vi "SubtractPolarVectors.vi"(10 "B":cluster{"Magnitude":dbl, "Direction":dbl}, 11 "A":cluster{"Magnitude":dbl, "Direction":dbl}) -> (3 "A-B":cluster{"Magnitude":dbl, "Direction":dbl})   [LabVIEW 2014]
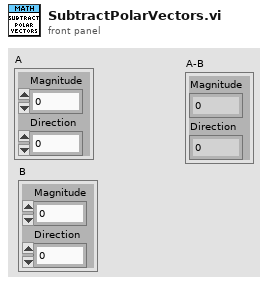
[diagram p1: front panel]
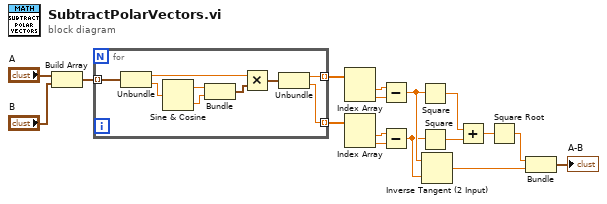
[diagram p0: block diagram]
diagram:
  n1 = Build Array("A", "B") -> (w15:cluster{"Magnitude":dbl, "Direction":dbl}[])
  n2 = for {
    tunnel: w15 -> [w26] mode=indexing
    tunnel: [w19] -> w14 mode=indexing
    tunnel: [w18] -> w13 mode=indexing
    n3 = Unbundle(w26) -> ("Magnitude"=w21:dbl, "Direction"=w25:dbl)
    n4 = Sine & Cosine(0:w25) -> (1:w23:dbl, 2:w24:dbl)
    n5 = Bundle(w23, w24) -> (w22:cluster{dbl, dbl})  [unwired: 1 in]
    n6 = Multiply(x=w21, y=w22) -> (x*y=w20:cluster{dbl, dbl})
    n7 = Unbundle(w20) -> (w19:dbl, w18:dbl)
  }
  n8 = Index Array(array=w14) -> (element #1=w11:dbl, element #2=w12:dbl)  [unwired: 2 in]
  n9 = Index Array(array=w13) -> (element #1=w9:dbl, element #2=w10:dbl)  [unwired: 2 in]
  n10 = Subtract(x=w11, y=w12) -> (x-y=w8:dbl)
  n11 = Subtract(x=w9, y=w10) -> (x-y=w7:dbl)
  n12 = Square(x=w8) -> (x^2=w5:dbl)
  n13 = Square(x=w7) -> (x^2=w6:dbl)
  n14 = Inverse Tangent (2 Input)(1:w7, 2:w8) -> (0:w2:dbl)
  n15 = Add(x=w5, y=w6) -> (x+y=w4:dbl)
  n16 = Square Root(x=w4) -> (sqrt(x)=w3:dbl)
  n17 = Bundle(w3, w2) -> (→"A-B":cluster{dbl, dbl})  [unwired: 1 in]
